vi "Vibration Sensors.vi"(8 "error in (no error)":errorcluster, 10 "Data Queue":refnum<queue>, 11 "Vibration Queue":refnum<queue>) -> (0 "error out":errorcluster)   [LabVIEW 2016]
uses:
  Message Format.ctl
  States.ctl
  <vilib>/DAQmx/read.llb/DAQmx Read (Analog 1D Wfm NChan NSamp).vi
  <vilib>/DAQmx/miscellaneous.llb/DAQmx Fill In Error Info.vi
  <resource>/objmgr/daqmx.rc
  <vilib>/ptbypt/NI_PtbyPt.lvlib
panel:
  out "step size (s)":dbl
  out "display duration (s)":dbl
  in  "STFT sample size":i32=512
  out "Spectral Density (dB)":dbl[][](graph)
  out "Spectrogram":dbl[][](graph)
  out "Raw Signal":waveform(dbl)(graph)
  in  "samples per step":i32=32
  in  "samples per FFT/window":i32=512
  out "sampling rate":dbl
  in  "samples per read block":i32=2560
  # "Vibration Sensors"
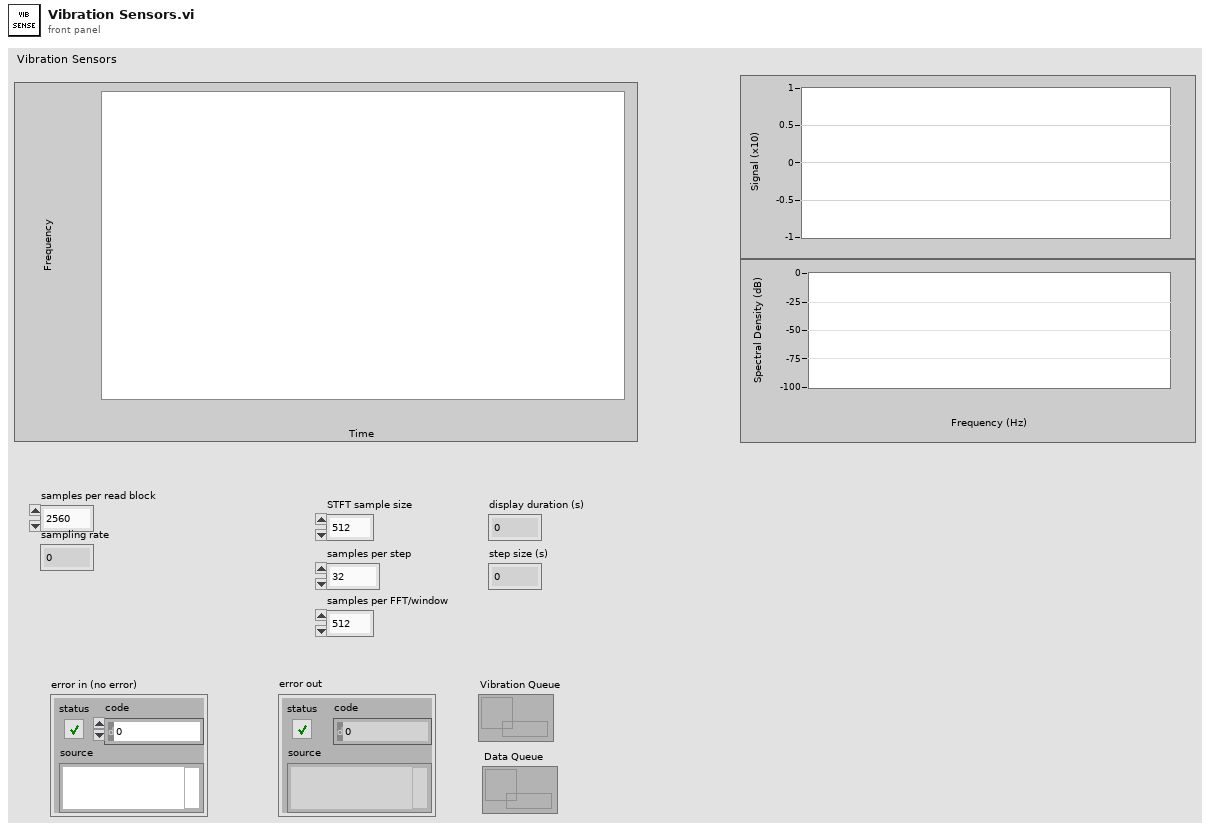
[diagram p1: front panel]
types:
  T1 = typedef "States.ctl" = enum16{"Initialize", "Running", "Exit"}
  T2 = typedef "Message Format.ctl" = cluster{"header":string, "data":variant}
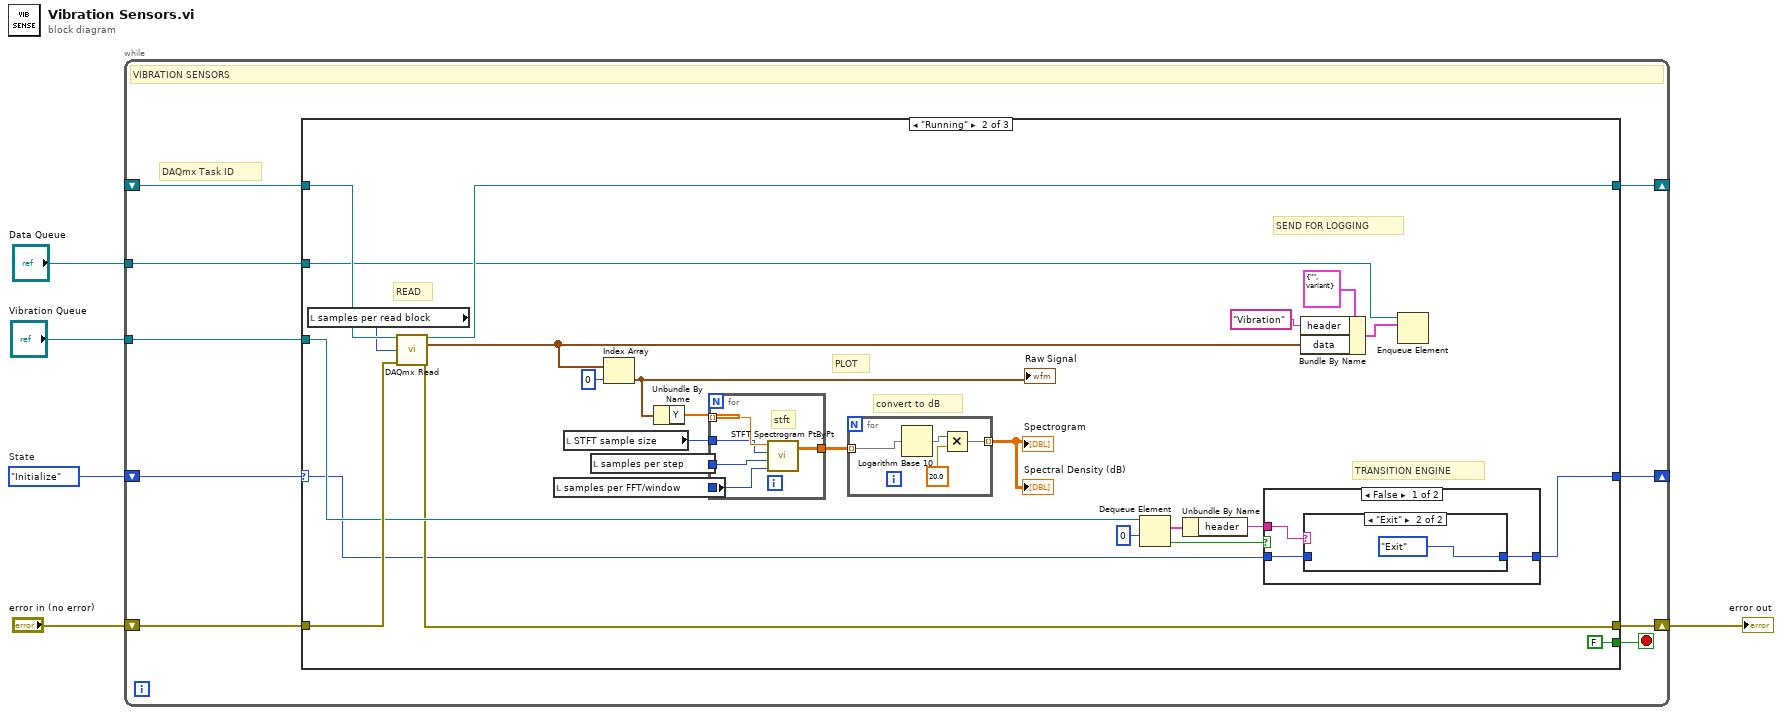
[diagram p0: block diagram]
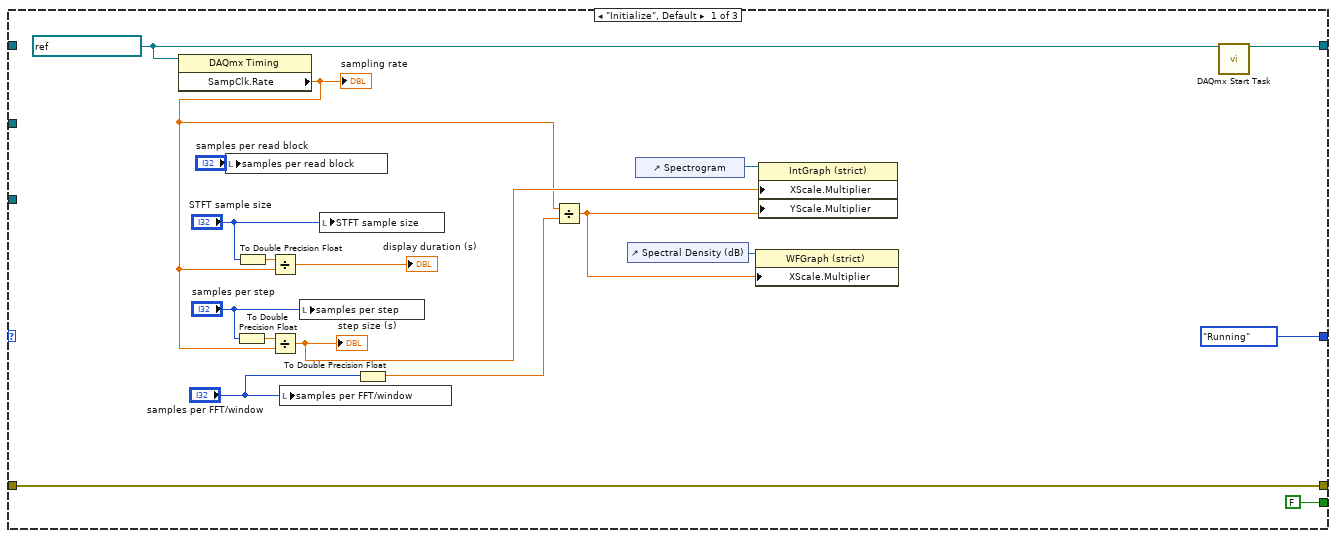
[diagram p2: hidden frame]
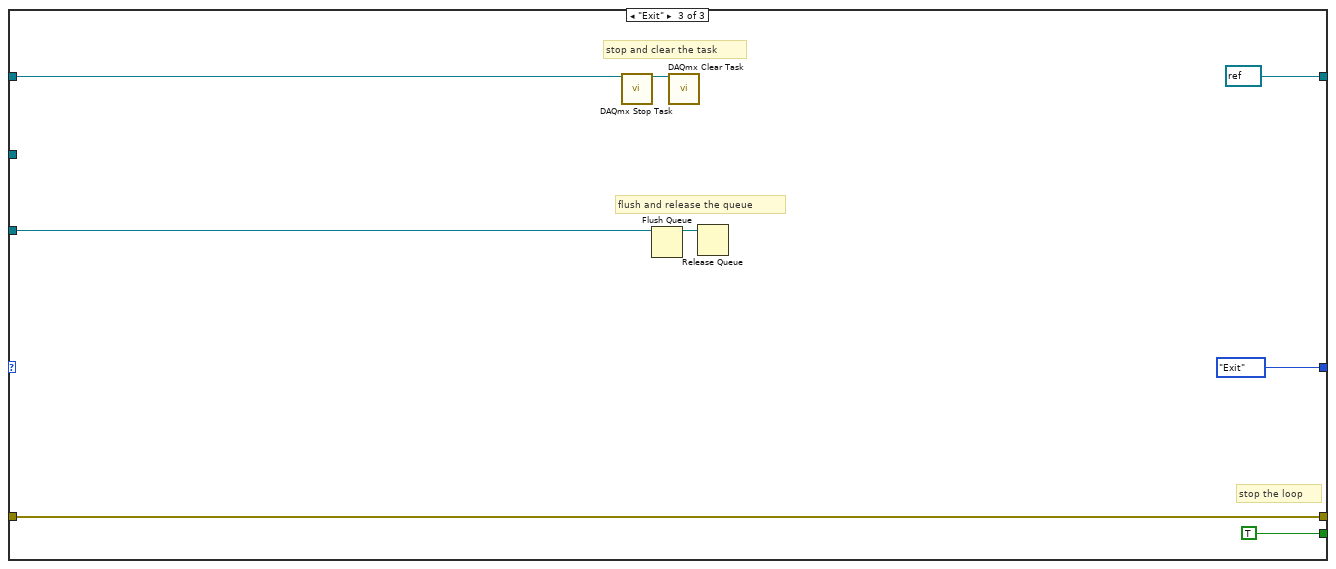
[diagram p5: hidden frame]
diagram:
  w3 = States."Initialize"  # State
  n1 = while {
    tunnel: "Vibration Queue" -> [w9]
    shift-right: [w14] -> w1
    shift-left: "error in (no error)" -> [w8]
    shift-right: [w13] -> _
    shift-left: _ -> [w12]
    tunnel: "Data Queue" -> [w11]
    shift-right: [w7] -> _
    shift-left: w3 -> [w10]
    stop <- w6 stop-if-true
    # "DAQmx Task ID"
    # "VIBRATION SENSORS"
    n2 = case shown="\"Running\"" w10 {
      selector: w10 -> [_ w37 _]
      tunnel: w8 -> [w17 w58 w75]
      tunnel: w9 -> [_ w40 w81]
      tunnel: [w17 w39 w75] -> w14
      tunnel: [w15 w55 refnum<k21> refnum ("task out")] -> w13
      tunnel: w12 -> [_ w57 w80]
      tunnel: w11 -> [_ w42 _]
      tunnel: [States."Running" ("State") w34 States."Exit" ("State")] -> w7
      tunnel: [FALSE FALSE TRUE] -> w6
      frame "Initialize", Default {
        w31 = refnum<k21> "VibrationTask" ("DAQmx Task Name")
        n3 = property class="DAQmx Timing"(reference=w31) -> ("SampClk.Rate"=w22:dbl)  [unwired: 1 in, 2 out]
        "sampling rate" <- w22
        n4 = local write "samples per read block"("samples per read block") -> ()
        n5 = To Double Precision Float(number="samples per step") -> (double precision float=w25:dbl)
        n6 = To Double Precision Float(number="STFT sample size") -> (double precision float=w27:dbl)
        n7 = Divide(x=w27, y=w22) -> (x/y=→"display duration (s)":dbl)
        n8 = Divide(x=w25, y=w22) -> (x/y=w23:dbl)
        "step size (s)" <- w23
        n9 = local write "samples per FFT/window"("samples per FFT/window") -> ()
        n10 = local write "samples per step"("samples per step") -> ()
        n11 = local write "STFT sample size"("STFT sample size") -> ()
        n12 = To Double Precision Float(number="samples per FFT/window") -> (double precision float=w16:dbl)
        n13 = Divide(x=w22, y=w16) -> (x/y=w20:dbl)
        n14 = control-ref of="Spectral Density (dB)"() -> (w29:refnum<vi>)
        n15 = control-ref of="Spectrogram"() -> (w30:refnum<vi>)
        n16 = property class="WFGraph (strict)"(reference=w29, "XScale.Multiplier"=w20) -> ()  [unwired: 1 in, 2 out]
        n17 = property on="Property Node" class="IntGraph (strict)"(reference=w30, "XScale.Multiplier"=w23, "YScale.Multiplier"=w20) -> ()  [unwired: 1 in, 2 out]
        n18 = call <vilib>:"DAQmx Start Task.vi"("task/channels in"=w31) -> ("task out"=w15:refnum<k21>)  [unwired: 13 in, 1 out]
      }
      frame "Running" {
        # "TRANSITION ENGINE"
        # "PLOT"
        # "convert to dB"
        # "SEND FOR LOGGING"
        # "READ"
        n19 = local read "samples per read block"() -> (w56:i32)
        n20 = call-poly <vilib>:"DAQmx Read.vi"("task/channels in"=w57, "number of samples per channel"=w56, "error in"=w58) -> ("task out"=w55:refnum<k21>, "data"=w43:waveform(dbl)[], "error out"=w39:errorcluster)  [unwired: 10 in]
        n21 = local read "samples per FFT/window"() -> (w53:i32)
        n22 = local read "STFT sample size"() -> (w54:i32)
        n23 = local read "samples per step"() -> (w50:i32)
        n24 = Index Array(array=w43, index=0) -> (element=w45:waveform(dbl))
        "Raw Signal" <- w45
        n25 = Unbundle By Name(w45) -> ("Y"=w44:dbl[])
        n26 = for {
          tunnel: w44 -> [w73] mode=indexing
          tunnel: w50 -> [w71]
          tunnel: w54 -> [w72]
          tunnel: w53 -> [w70]
          tunnel: [w69] -> w52
          # "stft"
          n27 = call <vilib>:"STFT Spectrogram PtByPt.vi"("window length"=w70, "time increment"=w71, "sample length"=w72, "x"=w73) -> ("STFT Spectrogram {X}"=w69:dbl[][])  [unwired: 2 in, 1 out]
        }
        n28 = for {
          tunnel: w52 -> [w68] mode=indexing
          tunnel: [w65] -> w51 mode=indexing
          n29 = Logarithm Base 10(1:w68) -> (0:w67:dbl[])
          n30 = Multiply(x=w67, y=20.0) -> (x*y=w65:dbl[])
        }
        "Spectrogram" <- w51
        "Spectral Density (dB)" <- w51
        n31 = Dequeue Element(queue=w40, timeout in ms (-1)=0) -> (element=w36:T2, timed out?=w38:bool)  [unwired: 1 in, 2 out]
        n32 = Unbundle By Name(w36) -> ("header"=w35:string)
        n33 = case shown="False" w38 {
          tunnel: w37 -> [w59 w64]
          tunnel: w35 -> [w61 _]
          tunnel: [w60 w64] -> w34
          frame False {
            n34 = case shown="\"Exit\"" w61 {
              tunnel: [w62 States."Exit" ("State")] -> w60
              tunnel: w59 -> [w62 _]
              frame "any other", Default {
              }
              frame "Exit" {
              }
            }
          }
          frame True {
          }
        }
        n35 = Bundle By Name(cluster=T2 {"header"="", "data"=variant} ("msg format"), "header"="Vibration", "data"=w43) -> (w47:T2)
        n36 = Enqueue Element(queue=w42, element=w47) -> ()  [unwired: 2 in, 3 out]
      }
      frame "Exit" {
        # "stop the loop"
        # "stop and clear the task"
        # "flush and release the queue"
        n37 = call <vilib>:"DAQmx Stop Task.vi"("task/channels in"=w80) -> ("task out"=w77:refnum<k21>)  [unwired: 13 in, 1 out]
        n38 = Flush Queue(queue=w81) -> (queue out=w74:refnum<queue>)  [unwired: 1 in, 2 out]
        n39 = call <vilib>:"DAQmx Clear Task.vi"("task in"=w77) -> ()  [unwired: 14 in, 1 out]
        n40 = Release Queue(queue=w74) -> ()  [unwired: 2 in, 3 out]
      }
    }
  }
  "error out" <- w1
